vi "CheckUpdatedSettings__LCR.vi"(8 "error in (no error)":errorcluster, 10 "Old State":T1={"Orientation"=0, "ActivePicture"={"image type"=0, "image depth"=0, "image"=[], "mask"=[], "colors"=[], "Rectangle"={"left"=0, "top"=0, "right"=0, "bottom"=0}}, "Pictures"={"Normal"={"image type"=0, "image depth"=0, "image"=[], "mask"=[], "colors"=[], "Rectangle"={"left"=0, "top"=0, "right"=0, "bottom"=0}}, "Hilite"={"image type"=0, "image depth"=0, "image"=[], "mask"=[], "colors"=[], "Rectangle"={"left"=0, "top"=0, "right"=0, "bottom"=0}}}, "Text"={"String"="", "Font"={"Font Name:"="", "Size"=0, "Strikeout?"=FALSE, "Italic?"=FALSE, "Underline?"=FALSE, "Outline?"=FALSE, "Shadow?"=FALSE, "Bold?"=FALSE}, "TextColor"=0}, "RunTimeSettings"={"Highlight"=FALSE, "ShowButton"=TRUE, "Behaviour"=enum."Switch when pressed", "React if disabled"=FALSE, "Nudge Button"=TRUE, "ShowButton on Hover"=FALSE, "Button Type"=enum."System"}, "Messages"=[], "Status"=0, "XControl Label"="", "Boolean Value"=FALSE} {"Status" format="%.0x"}, 11 "New State":T1={"Orientation"=0, "ActivePicture"={"image type"=0, "image depth"=0, "image"=[], "mask"=[], "colors"=[], "Rectangle"={"left"=0, "top"=0, "right"=0, "bottom"=0}}, "Pictures"={"Normal"={"image type"=0, "image depth"=0, "image"=[], "mask"=[], "colors"=[], "Rectangle"={"left"=0, "top"=0, "right"=0, "bottom"=0}}, "Hilite"={"image type"=0, "image depth"=0, "image"=[], "mask"=[], "colors"=[], "Rectangle"={"left"=0, "top"=0, "right"=0, "bottom"=0}}}, "Text"={"String"="", "Font"={"Font Name:"="", "Size"=0, "Strikeout?"=FALSE, "Italic?"=FALSE, "Underline?"=FALSE, "Outline?"=FALSE, "Shadow?"=FALSE, "Bold?"=FALSE}, "TextColor"=0}, "RunTimeSettings"={"Highlight"=FALSE, "ShowButton"=TRUE, "Behaviour"=enum."Switch when pressed", "React if disabled"=FALSE, "Nudge Button"=TRUE, "ShowButton on Hover"=FALSE, "Button Type"=enum."System"}, "Messages"=[], "Status"=0, "XControl Label"="", "Boolean Value"=FALSE} {"Status" format="%.0x"}) -> (0 "error out":errorcluster, 2 "State Out":T1={"Orientation"=0, "ActivePicture"={"image type"=0, "image depth"=0, "image"=[], "mask"=[], "colors"=[], "Rectangle"={"left"=0, "top"=0, "right"=0, "bottom"=0}}, "Pictures"={"Normal"={"image type"=0, "image depth"=0, "image"=[], "mask"=[], "colors"=[], "Rectangle"={"left"=0, "top"=0, "right"=0, "bottom"=0}}, "Hilite"={"image type"=0, "image depth"=0, "image"=[], "mask"=[], "colors"=[], "Rectangle"={"left"=0, "top"=0, "right"=0, "bottom"=0}}}, "Text"={"String"="", "Font"={"Font Name:"="", "Size"=0, "Strikeout?"=FALSE, "Italic?"=FALSE, "Underline?"=FALSE, "Outline?"=FALSE, "Shadow?"=FALSE, "Bold?"=FALSE}, "TextColor"=0}, "RunTimeSettings"={"Highlight"=FALSE, "ShowButton"=TRUE, "Behaviour"=enum."Switch when pressed", "React if disabled"=FALSE, "Nudge Button"=TRUE, "ShowButton on Hover"=FALSE, "Button Type"=enum."System"}, "Messages"=[], "Status"=0, "XControl Label"="", "Boolean Value"=FALSE} caption="State" {"Status" format="%.0x"})   [LabVIEW 2011, in "BooleanXControl__LCR.xctl"]
doc: "Compares the Old and New state of the BX and will trigger the Messages User event."
uses:
  BooleanXControl__LCR.xctl
  Abilities/BX.State__LCR.ctl
  Controls/BX.Orientation__LCR.ctl
  <vilib>/picture/picture.llb/imagedata.ctl
  Controls/BX.RTSettings__LCR.ctl
  Controls/BX.Behaviour__LCR.ctl
  Controls/BX.ButtonType__LCR.ctl
  Controls/BX.Message__LCR.ctl
  Controls/BX.Commands__LCR.ctl
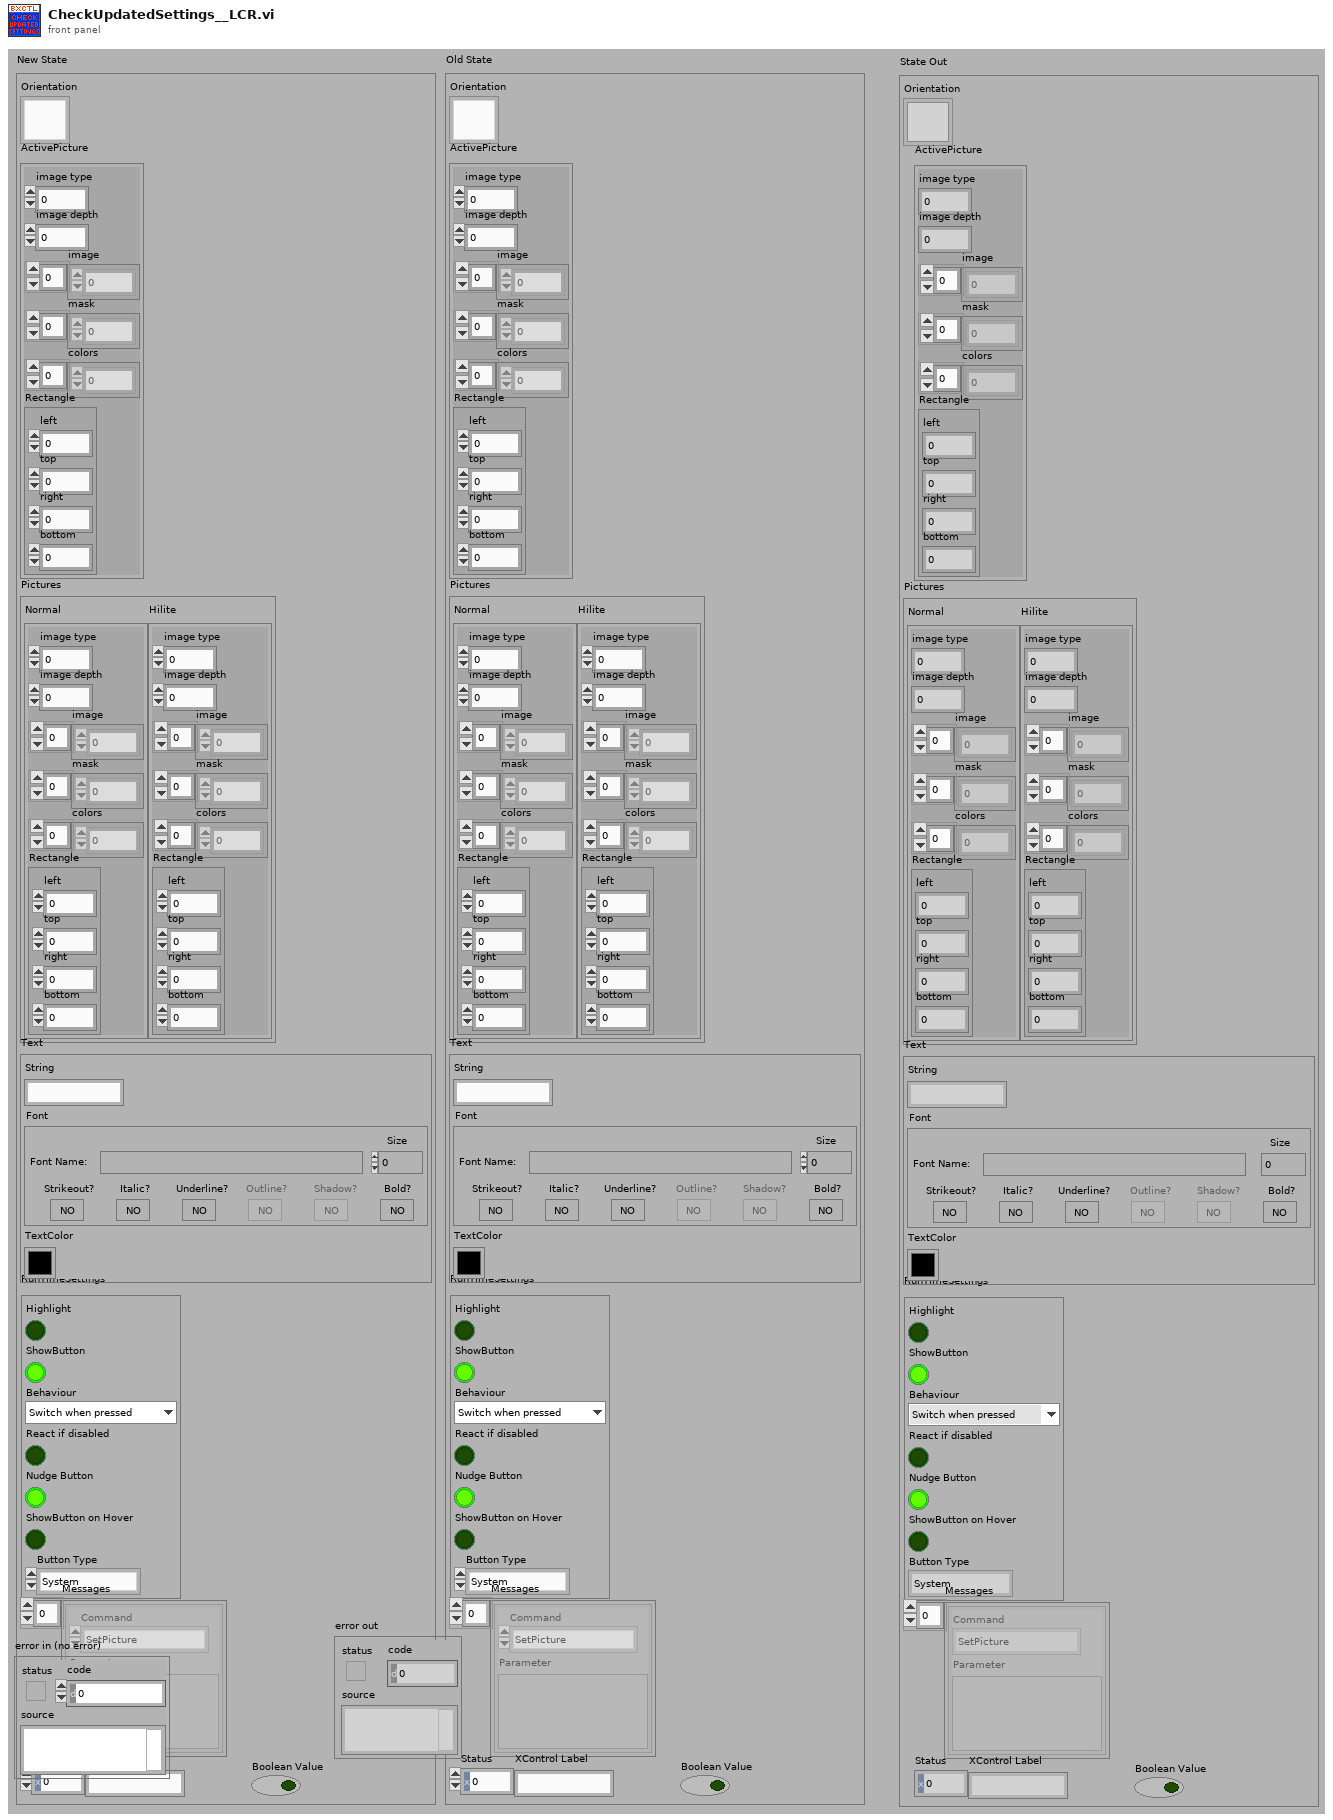
[diagram p1: front panel]
types:
  T1 = typedef "BooleanXControl__LCR.xctl/BX.State__LCR.ctl" = cluster{"Orientation":T2, "ActivePicture":T3, "Pictures":cluster{"Normal":T3, "Hilite":T3}, "Text":cluster{"String":string, "Font":cluster{"Font Name:":string, "Size":i16, "Strikeout?":bool, "Italic?":bool, "Underline?":bool, "Outline?":bool, "Shadow?":bool, "Bold?":bool}, "TextColor":u32}, "RunTimeSettings":T4, "Messages":T7[], "Status":u16, "XControl Label":string, "Boolean Value":bool}
  T2 = typedef "BooleanXControl__LCR.xctl/BX.Orientation__LCR.ctl" = u8
  T3 = typedef "imagedata.ctl" = cluster{"image type":i32, "image depth":i32, "image":u8[], "mask":u8[], "colors":u32[], "Rectangle":cluster{"left":i16, "top":i16, "right":i16, "bottom":i16}}
  T4 = typedef "BooleanXControl__LCR.xctl/BX.RTSettings__LCR.ctl" = cluster{"Highlight":bool, "ShowButton":bool, "Behaviour":T5, "React if disabled":bool, "Nudge Button":bool, "ShowButton on Hover":bool, "Button Type":T6}
  T5 = typedef "BooleanXControl__LCR.xctl/BX.Behaviour__LCR.ctl" = enum16{"Switch when pressed", "Switch when released", "Switch until released"}
  T6 = typedef "BooleanXControl__LCR.xctl/BX.ButtonType__LCR.ctl" = enum16{"System", "Modern", "Classic", "Decoration"}
  T7 = typedef "BooleanXControl__LCR.xctl/BX.Message__LCR.ctl" = cluster{"Command":T8, "Parameter":variant}
  T8 = typedef "BooleanXControl__LCR.xctl/BX.Commands__LCR.ctl" = enum16{"None", "SetPicture", "SetFont", "SetText", "SetOrientation", "Redraw", "SetTextColor", "SetRTSettings", "MultipleUpdate", "RT.Button", "RT.Hilite", "RT.Behaviour", "RT.Disabled", "ShowGUI", "RT.Nudge", "RT.Hover", "RT.ButtonType"}
  T9 = cluster{"Orientation":bool, "ActivePicture":cluster{"image type":bool, "image depth":bool, "image":bool[], "mask":bool[], "colors":bool[], "Rectangle":cluster{"left":bool, "top":bool, "right":bool, "bottom":bool}}, "Pictures":cluster{"Normal":cluster{"image type":bool, "image depth":bool, "image":bool[], "mask":bool[], "colors":bool[], "Rectangle":cluster{"left":bool, "top":bool, "right":bool, "bottom":bool}}, "Hilite":cluster{"image type":bool, "image depth":bool, "image":bool[], "mask":bool[], "colors":bool[], "Rectangle":cluster{"left":bool, "top":bool, "right":bool, "bottom":bool}}}, "Text":cluster{"String":bool, "Font":cluster{"Font Name:":bool, "Size":bool, "Strikeout?":bool, "Italic?":bool, "Underline?":bool, "Outline?":bool, "Shadow?":bool, "Bold?":bool}, "TextColor":bool}, "RunTimeSettings":cluster{"Highlight":bool, "ShowButton":bool, "Behaviour":bool, "React if disabled":bool, "Nudge Button":bool, "ShowButton on Hover":bool, "Button Type":bool}, "Messages":cluster{"Command":bool, "Parameter":bool}[], "Status":bool, "XControl Label":bool, "Boolean Value":bool}
  T10 = cluster{"Font Name:":string, "Size":i16, "Strikeout?":bool, "Italic?":bool, "Underline?":bool, "Outline?":bool, "Shadow?":bool, "Bold?":bool}
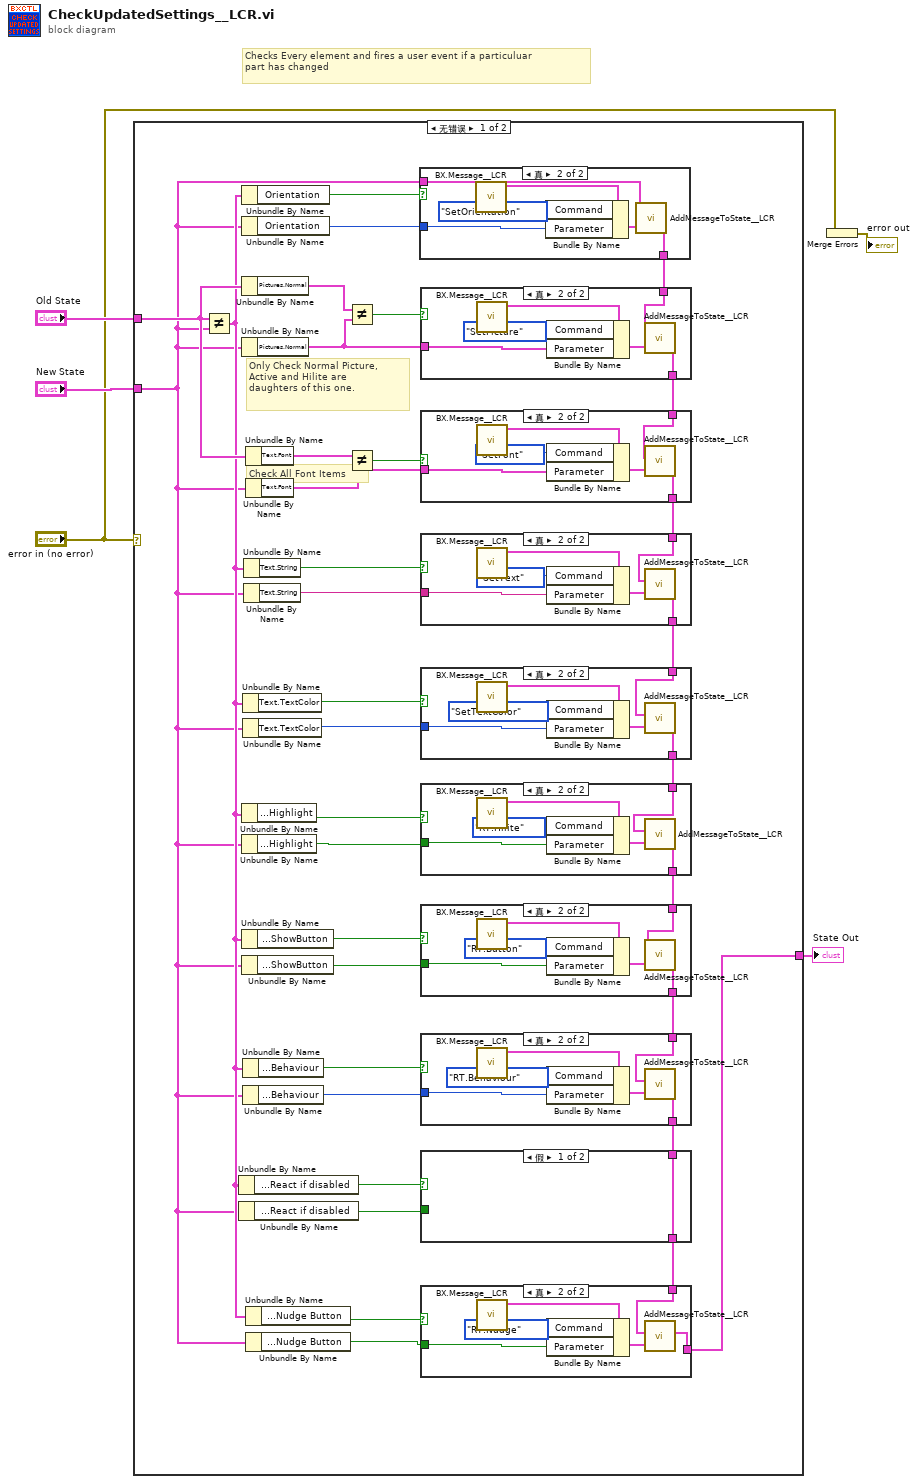
[diagram p0: block diagram]
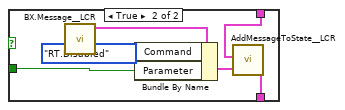
[diagram p3: hidden frame]
diagram:
  # "Checks Every element and fires a user event if a particuluar\npart has changed"
  n1 = case shown="无错误" "error in (no error)" {
    tunnel: "Old State" -> [w24 _]
    tunnel: "New State" -> [w8 w111]
    tunnel: [w10 w111] -> w1
    frame No Error {
      # "Only Check Normal Picture,\nActive and Hilite are \ndaughters of this one."
      # "Check All Font Items"
      n2 = Not Equal?(x=w24, y=w8) -> (x != y?=w9:T9)
      n3 = Unbundle By Name(w9) -> ("RunTimeSettings.React if disabled"=w22:bool)
      n4 = Unbundle By Name(w8) -> ("RunTimeSettings.React if disabled"=w25:bool)
      n5 = Unbundle By Name(w9) -> ("Orientation"=w39:bool)
      n6 = Unbundle By Name(w8) -> ("Orientation"=w40:T2)
      n7 = Unbundle By Name(w24) -> ("Pictures.Normal"=w37:T3)
      n8 = Unbundle By Name(w8) -> ("Pictures.Normal"=w38:T3)
      n9 = Unbundle By Name(w9) -> ("RunTimeSettings.Highlight"=w23:bool)
      n10 = Unbundle By Name(w8) -> ("RunTimeSettings.Highlight"=w28:bool)
      n11 = Unbundle By Name(w9) -> ("RunTimeSettings.ShowButton"=w20:bool)
      n12 = Unbundle By Name(w8) -> ("RunTimeSettings.ShowButton"=w27:bool)
      n13 = Unbundle By Name(w9) -> ("Text.TextColor"=w30:bool)
      n14 = Unbundle By Name(w8) -> ("Text.TextColor"=w29:u32)
      n15 = Unbundle By Name(w9) -> ("RunTimeSettings.Behaviour"=w21:bool)
      n16 = Unbundle By Name(w8) -> ("RunTimeSettings.Behaviour"=w26:T5)
      n17 = Unbundle By Name(w9) -> ("Text.String"=w32:bool)
      n18 = Unbundle By Name(w8) -> ("Text.String"=w31:string)
      n19 = Unbundle By Name(w24) -> ("Text.Font"=w35:T10)
      n20 = Unbundle By Name(w8) -> ("Text.Font"=w34:T10)
      n21 = Unbundle By Name(w9) -> ("RunTimeSettings.Nudge Button"=w7:bool)
      n22 = Unbundle By Name(w8) -> ("RunTimeSettings.Nudge Button"=w6:bool)
      n23 = Not Equal?(x=w37, y=w38) -> (x != y?=w36:bool)
      n24 = Not Equal?(x=w35, y=w34) -> (x != y?=w33:bool)
      n25 = case shown="真" w39 {
        tunnel: w40 -> [_ w108]
        tunnel: [w104 w106] -> w19
        tunnel: w8 -> [w104 w105]
        frame False {
        }
        frame True {
          n26 = call "BX.Message__LCR.vi"() -> ("Messages"=w109:T7)  [unwired: 11 in]
          n27 = Bundle By Name(cluster=w109, "Command"=BX.Commands__LCR."SetOrientation", "Parameter"=w108) -> (w107:T7)
          n28 = call "AddMessageToState__LCR.vi"("Message"=w107, "State In"=w105) -> ("State Out"=w106:T1)  [unwired: 9 in]
        }
      }
      n29 = case shown="真" w36 {
        tunnel: w38 -> [_ w101]
        tunnel: w19 -> [w97 w100]
        tunnel: [w97 w98] -> w18
        frame False {
        }
        frame True {
          n30 = call "BX.Message__LCR.vi"() -> ("Messages"=w102:T7)  [unwired: 11 in]
          n31 = Bundle By Name(cluster=w102, "Command"=BX.Commands__LCR."SetPicture", "Parameter"=w101) -> (w99:T7)
          n32 = call "AddMessageToState__LCR.vi"("Message"=w99, "State In"=w100) -> ("State Out"=w98:T1)  [unwired: 9 in]
        }
      }
      n33 = case shown="真" w33 {
        tunnel: w34 -> [_ w94]
        tunnel: w18 -> [w90 w93]
        tunnel: [w90 w91] -> w17
        frame False {
        }
        frame True {
          n34 = call "BX.Message__LCR.vi"() -> ("Messages"=w95:T7)  [unwired: 11 in]
          n35 = Bundle By Name(cluster=w95, "Command"=BX.Commands__LCR."SetFont", "Parameter"=w94) -> (w92:T7)
          n36 = call "AddMessageToState__LCR.vi"("Message"=w92, "State In"=w93) -> ("State Out"=w91:T1)  [unwired: 9 in]
        }
      }
      n37 = case shown="真" w32 {
        tunnel: w31 -> [_ w87]
        tunnel: w17 -> [w83 w86]
        tunnel: [w83 w84] -> w16
        frame False {
        }
        frame True {
          n38 = call "BX.Message__LCR.vi"() -> ("Messages"=w88:T7)  [unwired: 11 in]
          n39 = Bundle By Name(cluster=w88, "Command"=BX.Commands__LCR."SetText", "Parameter"=w87) -> (w85:T7)
          n40 = call "AddMessageToState__LCR.vi"("Message"=w85, "State In"=w86) -> ("State Out"=w84:T1)  [unwired: 9 in]
        }
      }
      n41 = case shown="真" w30 {
        tunnel: w29 -> [_ w80]
        tunnel: w16 -> [w76 w79]
        tunnel: [w76 w77] -> w15
        frame False {
        }
        frame True {
          n42 = call "BX.Message__LCR.vi"() -> ("Messages"=w81:T7)  [unwired: 11 in]
          n43 = Bundle By Name(cluster=w81, "Command"=BX.Commands__LCR."SetTextColor", "Parameter"=w80) -> (w78:T7)
          n44 = call "AddMessageToState__LCR.vi"("Message"=w78, "State In"=w79) -> ("State Out"=w77:T1)  [unwired: 9 in]
        }
      }
      n45 = case shown="真" w23 {
        tunnel: w28 -> [_ w73]
        tunnel: w15 -> [w69 w72]
        tunnel: [w69 w70] -> w14
        frame False {
        }
        frame True {
          n46 = call "BX.Message__LCR.vi"() -> ("Messages"=w74:T7)  [unwired: 11 in]
          n47 = Bundle By Name(cluster=w74, "Command"=BX.Commands__LCR."RT.Hilite", "Parameter"=w73) -> (w71:T7)
          n48 = call "AddMessageToState__LCR.vi"("Message"=w71, "State In"=w72) -> ("State Out"=w70:T1)  [unwired: 9 in]
        }
      }
      n49 = case shown="真" w20 {
        tunnel: w27 -> [_ w66]
        tunnel: w14 -> [w62 w65]
        tunnel: [w62 w63] -> w13
        frame False {
        }
        frame True {
          n50 = call "BX.Message__LCR.vi"() -> ("Messages"=w67:T7)  [unwired: 11 in]
          n51 = Bundle By Name(cluster=w67, "Command"=BX.Commands__LCR."RT.Button", "Parameter"=w66) -> (w64:T7)
          n52 = call "AddMessageToState__LCR.vi"("Message"=w64, "State In"=w65) -> ("State Out"=w63:T1)  [unwired: 9 in]
        }
      }
      n53 = case shown="真" w21 {
        tunnel: w26 -> [_ w59]
        tunnel: w13 -> [w55 w58]
        tunnel: [w55 w56] -> w12
        frame False {
        }
        frame True {
          n54 = call "BX.Message__LCR.vi"() -> ("Messages"=w60:T7)  [unwired: 11 in]
          n55 = Bundle By Name(cluster=w60, "Command"=BX.Commands__LCR."RT.Behaviour", "Parameter"=w59) -> (w57:T7)
          n56 = call "AddMessageToState__LCR.vi"("Message"=w57, "State In"=w58) -> ("State Out"=w56:T1)  [unwired: 9 in]
        }
      }
      n57 = case shown="假" w22 {
        tunnel: w25 -> [_ w52]
        tunnel: w12 -> [w48 w51]
        tunnel: [w48 w49] -> w11
        frame False {
        }
        frame True {
          n58 = call "BX.Message__LCR.vi"() -> ("Messages"=w53:T7)  [unwired: 11 in]
          n59 = Bundle By Name(cluster=w53, "Command"=BX.Commands__LCR."RT.Disabled", "Parameter"=w52) -> (w50:T7)
          n60 = call "AddMessageToState__LCR.vi"("Message"=w50, "State In"=w51) -> ("State Out"=w49:T1)  [unwired: 9 in]
        }
      }
      n61 = case shown="真" w7 {
        tunnel: w6 -> [_ w45]
        tunnel: [w41 w44] -> w10
        tunnel: w11 -> [w41 w43]
        frame False {
        }
        frame True {
          n62 = call "BX.Message__LCR.vi"() -> ("Messages"=w46:T7)  [unwired: 11 in]
          n63 = Bundle By Name(cluster=w46, "Command"=BX.Commands__LCR."RT.Nudge", "Parameter"=w45) -> (w42:T7)
          n64 = call "AddMessageToState__LCR.vi"("Message"=w42, "State In"=w43) -> ("State Out"=w44:T1)  [unwired: 9 in]
        }
      }
    }
    frame Error {
    }
  }
  "State Out" <- w1
  n65 = Merge Errors("error in (no error)") -> (→"error out":errorcluster)
